vi "emballage affiche le contenu du carton_MEDIC.vi"(1 "Tableau historique":string[][](array[string])=[["MK0228606ARXA2199", "24.02.2006 11:58", "AFA", "5401/04", "1", "200"], ["MK0228606ARXA2177", "24.02.2006 12:00", "AFA", "5401/04", "1", "200"], ["MK0228606ARXA2178", "24.02.2006 12:00", "AFA", "5401/04", "1", "200"], ["MK0228606ARXA2198", "24.02.2006 12:12", "AFA", "5401/04", "1", "200"], ["MK0228606ARXA2197", "24.02.2006 12:12", "AFA", "5401/04", "1", "200"], ["MK0228606ARXA2196", "24.02.2006 12:13", "AFA", "5401/04", "1", "200"], ["MK0228606ARXA2195", "24.02.2006 12:13", "AFA", "5401/04", "1", "200"], ["MK0228606ARXA2176", "24.02.2006 12:13", "AFA", "5401/04", "1", "200"], ["MK0228606ARXA2194", "24.02.2006 12:13", "AFA", "5401/04", "1", "200"], ["MK0228606ARXA2193", "24.02.2006 12:13", "AFA", "5401/04", "1", "200"], ["MK0228606ARXA2175", "24.02.2006 12:14", "AFA", "5401/04", "1", "200"], ["MK0228606ARXA2171", "24.02.2006 12:14", "AFA", "5401/04", "1", "200"], ["MK0228606ARXA2174", "24.02.2006 12:14", "AFA", "5401/04", "1", "200"], ["MK0228606ARXA2173", "24.02.2006 12:14", "AFA", "5401/04", "1", "200"], ["MK0228606ARXA2172", "24.02.2006 12:14", "AFA", "5401/04", "1", "200"], ["MK0228606ARXA2192", "24.02.2006 12:14", "AFA", "5401/04", "1", "200"], ["MK0228606ARXA2191", "24.02.2006 12:14", "AFA", "5401/04", "1", "200"], ["MK0228606ARXA2190", "24.02.2006 12:14", "AFA", "5401/04", "1", "200"], ["MK0228606ARXA2189", "24.02.2006 12:15", "AFA", "5401/04", "1", "200"], ["MK0228606ARXA2188", "24.02.2006 12:15", "AFA", "5401/04", "1", "200"], ["MK0228606ARXB4259", "09.03.2006 17:40", "AYU", "5401/04-03.03", "5", "300"], ["MK0228606ARXB4258", "09.03.2006 17:40", "AYU", "5401/04-03.03", "5", "300"], ["MK0228606ARXB4257", "09.03.2006 17:40", "AYU", "5401/04-03.03", "5", "300"], ["MK0228606ARXB4256", "09.03.2006 17:39", "AYU", "5401/04-03.03", "5", "300"], ["MK0228606ARXB4255", "09.03.2006 17:39", "AYU", "5401/04-03.03", "5", "300"], ["MK0228606ARXB4254", "09.03.2006 17:39", "AYU", "5401/04-03.03", "5", "300"], ["MK0228606ARXB4253", "09.03.2006 17:39", "AYU", "5401/04-03.03", "5", "300"], ["MK0228606ARXB4252", "09.03.2006 17:39", "AYU", "5401/04-03.03", "5", "300"], ["MK0228606ARXB4251", "09.03.2006 17:39", "AYU", "5401/04-03.03", "5", "300"], ["MK0228606ARXB4250", "09.03.2006 17:39", "AYU", "5401/04-03.03", "5", "300"], ["MK0228606ARXB4249", "09.03.2006 17:39", "AYU", "5401/04-03.03", "5", "300"], ["MK0228606ARXB4248", "09.03.2006 17:39", "AYU", "5401/04-03.03", "5", "300"], ["MK0228606ARXB4247", "09.03.2006 17:39", "AYU", "5401/04-03.03", "5", "300"], ["MK0228606ARXB4246", "09.03.2006 17:39", "AYU", "5401/04-03.03", "5", "300"], ["MK0228606ARXB4245", "09.03.2006 17:38", "AYU", "5401/04-03.03", "5", "300"], ["MK0228606ARXB4244", "09.03.2006 17:38", "AYU", "5401/04-03.03", "5", "300"], ["MK0228606ARXB4243", "09.03.2006 17:38", "AYU", "5401/04-03.03", "5", "300"], ["MK0228606ARXB4242", "09.03.2006 17:38", "AYU", "5401/04-03.03", "5", "300"], ["MK0228606ARXB4241", "09.03.2006 17:38", "AYU", "5401/04-03.03", "5", "300"], ["MK0228606ARXB4240", "09.03.2006 17:38", "AYU", "5401/04-03.03", "5", "300"], ["MK0228606ARXB4239", "09.03.2006 17:33", "AYU", "5401/04-03.03", "4", "300"], ["MK0228606ARXB4238", "09.03.2006 17:32", "AYU", "5401/04-03.03", "4", "300"], ["MK0228606ARXB4237", "09.03.2006 17:32", "AYU", "5401/04-03.03", "4", "300"], ["MK0228606ARXB4236", "09.03.2006 17:32", "AYU", "5401/04-03.03", "4", "300"], ["MK0228606ARXB4235", "09.03.2006 17:32", "AYU", "5401/04-03.03", "4", "300"], ["MK0228606ARXB4234", "09.03.2006 17:32", "AYU", "5401/04-03.03", "4", "300"], ["MK0228606ARXB4233", "09.03.2006 17:32", "AYU", "5401/04-03.03", "4", "300"], ["MK0228606ARXB4232", "09.03.2006 17:32", "AYU", "5401/04-03.03", "4", "300"], ["MK0228606ARXB4231", "09.03.2006 17:31", "AYU", "5401/04-03.03", "4", "300"], ["MK0228606ARXB4230", "09.03.2006 17:31", "AYU", "5401/04-03.03", "4", "300"], ["MK0228606ARXB4229", "09.03.2006 17:31", "AYU", "5401/04-03.03", "4", "300"], ["MK0228606ARXB4228", "09.03.2006 17:31", "AYU", "5401/04-03.03", "4", "300"], ["MK0228606ARXB4227", "09.03.2006 17:31", "AYU", "5401/04-03.03", "4", "300"], ["MK0228606ARXB4226", "09.03.2006 17:31", "AYU", "5401/04-03.03", "4", "300"], ["MK0228606ARXB4225", "09.03.2006 17:30", "AYU", "5401/04-03.03", "4", "300"], ["MK0228606ARXB4224", "09.03.2006 17:30", "AYU", "5401/04-03.03", "4", "300"], ["MK0228606ARXB4223", "09.03.2006 17:30", "AYU", "5401/04-03.03", "4", "300"], ["MK0228606ARXB4222", "09.03.2006 17:30", "AYU", "5401/04-03.03", "4", "300"], ["MK0228606ARXB4221", "09.03.2006 17:30", "AYU", "5401/04-03.03", "4", "300"], ["MK0228606ARXB4220", "09.03.2006 17:30", "AYU", "5401/04-03.03", "4", "300"], ["MK0228606ARXB4219", "09.03.2006 17:24", "AYU", "5401/04-03.03", "3", "300"], ["MK0228606ARXB4218", "09.03.2006 17:23", "AYU", "5401/04-03.03", "3", "300"], ["MK0228606ARXB4217", "09.03.2006 17:23", "AYU", "5401/04-03.03", "3", "300"], ["MK0228606ARXB4216", "09.03.2006 17:23", "AYU", "5401/04-03.03", "3", "300"], ["MK0228606ARXB4215", "09.03.2006 17:23", "AYU", "5401/04-03.03", "3", "300"], ["MK0228606ARXB4214", "09.03.2006 17:23", "AYU", "5401/04-03.03", "3", "300"], ["MK0228606ARXB4213", "09.03.2006 17:23", "AYU", "5401/04-03.03", "3", "300"], ["MK0228606ARXB4212", "09.03.2006 17:22", "AYU", "5401/04-03.03", "3", "300"], ["MK0228606ARXB4211", "09.03.2006 17:21", "AYU", "5401/04-03.03", "3", "300"], ["MK0228606ARXB4210", "09.03.2006 17:21", "AYU", "5401/04-03.03", "3", "300"], ["MK0228606ARXB4209", "09.03.2006 17:21", "AYU", "5401/04-03.03", "3", "300"], ["MK0228606ARXB4208", "09.03.2006 17:20", "AYU", "5401/04-03.03", "3", "300"], ["MK0228606ARXB4207", "09.03.2006 17:20", "AYU", "5401/04-03.03", "3", "300"], ["MK0228606ARXB4206", "09.03.2006 17:20", "AYU", "5401/04-03.03", "3", "300"], ["MK0228606ARXB4205", "09.03.2006 17:20", "AYU", "5401/04-03.03", "3", "300"], ["MK0228606ARXB4204", "09.03.2006 17:20", "AYU", "5401/04-03.03", "3", "300"], ["MK0228606ARXB4203", "09.03.2006 17:20", "AYU", "5401/04-03.03", "3", "300"], ["MK0228606ARXB4202", "09.03.2006 17:19", "AYU", "5401/04-03.03", "3", "300"], ["MK0228606ARXB4201", "09.03.2006 17:19", "AYU", "5401/04-03.03", "3", "300"], ["MK0228606ARXB4200", "09.03.2006 17:18", "AYU", "5401/04-03.03", "3", "300"], ["MK0228606ARXB4199", "09.03.2006 17:12", "AYU", "5401/04-03.03", "2", "300"], ["MK0228606ARXB4198", "09.03.2006 17:11", "AYU", "5401/04-03.03", "2", "300"], ["MK0228606ARXB4197", "09.03.2006 17:11", "AYU", "5401/04-03.03", "2", "300"], ["MK0228606ARXB4196", "09.03.2006 17:11", "AYU", "5401/04-03.03", "2", "300"], ["MK0228606ARXB4195", "09.03.2006 17:11", "AYU", "5401/04-03.03", "2", "300"], ["MK0228606ARXB4194", "09.03.2006 17:11", "AYU", "5401/04-03.03", "2", "300"], ["MK0228606ARXB4193", "09.03.2006 17:11", "AYU", "5401/04-03.03", "2", "300"], ["MK0228606ARXB4192", "09.03.2006 17:10", "AYU", "5401/04-03.03", "2", "300"], ["MK0228606ARXB4191", "09.03.2006 17:10", "AYU", "5401/04-03.03", "2", "300"], ["MK0228606ARXB4190", "09.03.2006 17:10", "AYU", "5401/04-03.03", "2", "300"], ["MK0228606ARXB4189", "09.03.2006 17:10", "AYU", "5401/04-03.03", "2", "300"], ["MK0228606ARXB4188", "09.03.2006 17:10", "AYU", "5401/04-03.03", "2", "300"], ["MK0228606ARXB4187", "09.03.2006 17:10", "AYU", "5401/04-03.03", "2", "300"], ["MK0228606ARXB4186", "09.03.2006 17:10", "AYU", "5401/04-03.03", "2", "300"], ["MK0228606ARXB4185", "09.03.2006 17:10", "AYU", "5401/04-03.03", "2", "300"], ["MK0228606ARXB4184", "09.03.2006 17:09", "AYU", "5401/04-03.03", "2", "300"], ["MK0228606ARXB4183", "09.03.2006 17:09", "AYU", "5401/04-03.03", "2", "300"], ["MK0228606ARXB4182", "09.03.2006 17:09", "AYU", "5401/04-03.03", "2", "300"], ["MK0228606ARXB4181", "09.03.2006 17:08", "AYU", "5401/04-03.03", "2", "300"], ["MK0228606ARXB4180", "09.03.2006 17:08", "AYU", "5401/04-03.03", "2", "300"], ["MK0228606ARXB4179", "09.03.2006 17:01", "AYU", "5401/04-03.03", "1", "300"], ["MK0228606ARXB4178", "09.03.2006 17:01", "AYU", "5401/04-03.03", "1", "300"], ["MK0228606ARXB4177", "09.03.2006 17:01", "AYU", "5401/04-03.03", "1", "300"], ["MK0228606ARXB4176", "09.03.2006 17:01", "AYU", "5401/04-03.03", "1", "300"], ["MK0228606ARXB4175", "09.03.2006 17:00", "AYU", "5401/04-03.03", "1", "300"], ["MK0228606ARXB4174", "09.03.2006 17:00", "AYU", "5401/04-03.03", "1", "300"], ["MK0228606ARXB4173", "09.03.2006 17:00", "AYU", "5401/04-03.03", "1", "300"], ["MK0228606ARXB4172", "09.03.2006 17:00", "AYU", "5401/04-03.03", "1", "300"], ["MK0228606ARXB4171", "09.03.2006 17:00", "AYU", "5401/04-03.03", "1", "300"], ["MK0228606ARXB4170", "09.03.2006 16:57", "AYU", "5401/04-03.03", "1", "300"], ["MK0228606ARXB4169", "09.03.2006 16:57", "AYU", "5401/04-03.03", "1", "300"], ["MK0228606ARXB4168", "09.03.2006 16:56", "AYU", "5401/04-03.03", "1", "300"], ["MK0228606ARXB4167", "09.03.2006 16:56", "AYU", "5401/04-03.03", "1", "300"], ["MK0228606ARXB4166", "09.03.2006 16:56", "AYU", "5401/04-03.03", "1", "300"], ["MK0228606ARXB4165", "09.03.2006 16:55", "AYU", "5401/04-03.03", "1", "300"], ["MK0228606ARXB4164", "09.03.2006 16:55", "AYU", "5401/04-03.03", "1", "300"], ["MK0228606ARXB4163", "09.03.2006 16:55", "AYU", "5401/04-03.03", "1", "300"], ["MK0228606ARXB4162", "09.03.2006 16:54", "AYU", "5401/04-03.03", "1", "300"], ["MK0228606ARXB4161", "09.03.2006 16:54", "AYU", "5401/04-03.03", "1", "300"], ["MK0228606ARXB4160", "09.03.2006 16:52", "AYU", "5401/04-03.03", "1", "300"], ["MK0228606ARXB4158", "10.03.2006 08:35", "AYU", "5401/04-03.03", "1", "300"], ["MK0228606ARXB4159", "10.03.2006 08:34", "AYU", "5401/04-03.03", "1", "300"]], 2 "chaîne 2D emballage en cours":string) -> ()   [LabVIEW 2020]
panel:
  in  "Tableau":string[](array[string])
  in  "quitter":bool
  out "Piéces dans le carton":i32(listbox)
  out "Numéro de la commande :":string
  in  "numéro du carton :":i16
  # "(si rien : prend la liste en cours d'emballage)"
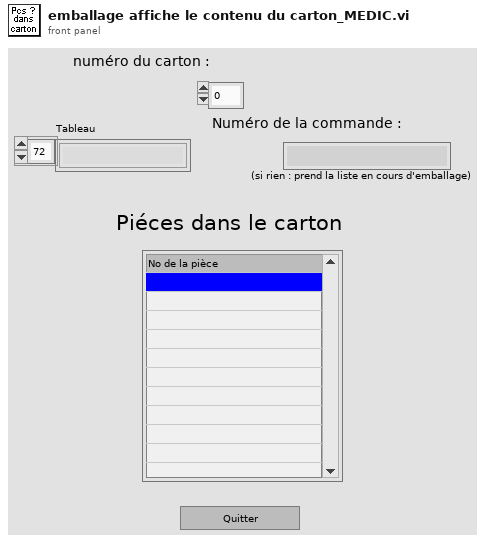
[diagram p1: front panel]
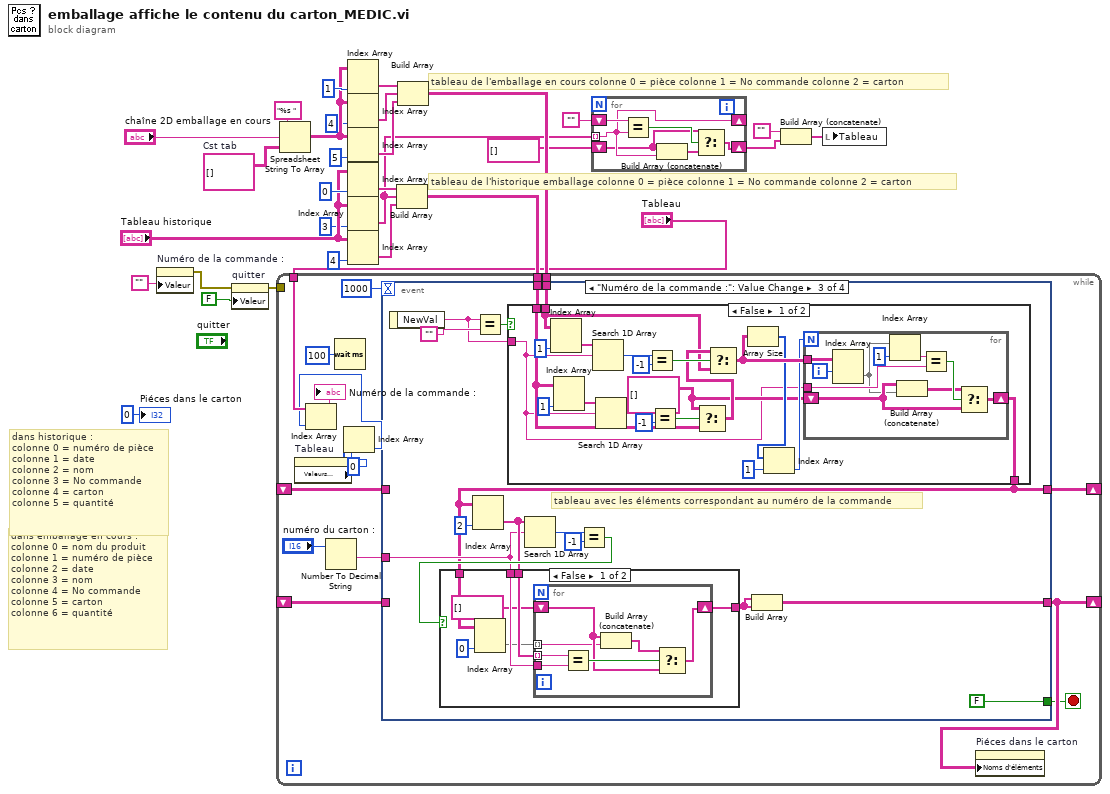
[diagram p0: block diagram]
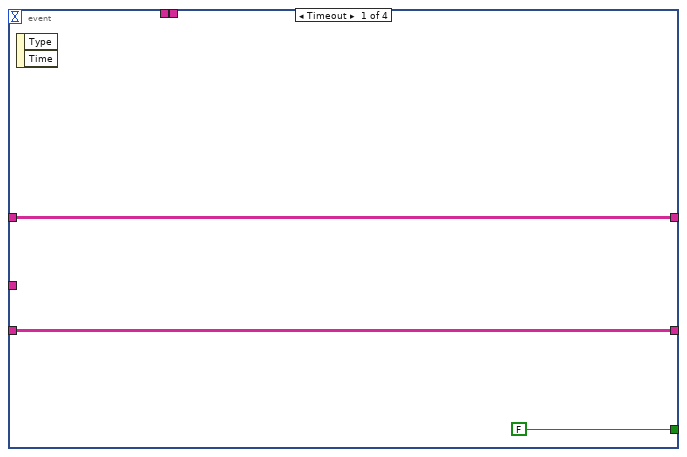
[diagram p2: hidden frame]
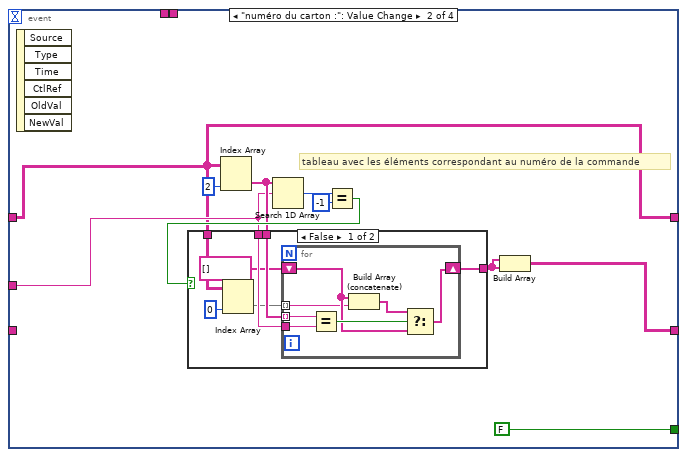
[diagram p3: hidden frame]
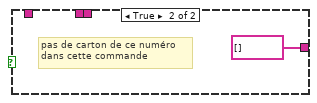
[diagram p4: hidden frame]
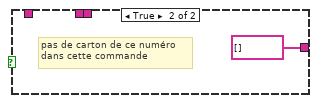
[diagram p5: hidden frame]
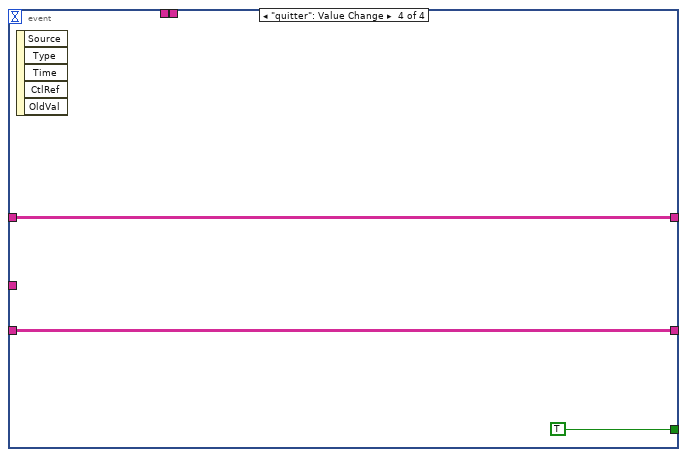
[diagram p7: hidden frame]
diagram:
  w25 = string[][] []  # Cst tab
  # "tableau de l'historique emballage colonne 0 = pièce colonne 1 = No commande colonne 2 = carton"
  # "tableau de l'emballage en cours colonne 0 = pièce colonne 1 = No commande colonne 2 = carton"
  # "dans emballage en cours :\ncolonne 0 = nom du produit\ncolonne 1 = numéro de pièce\ncolonne 2 = date\ncolonne 3 = nom\ncolonne 4 = No commande\ncolonne 5 = carton\ncolonne 6 = quantité"
  # "dans historique :\ncolonne 0 = numéro de pièce\ncolonne 1 = date\ncolonne 2 = nom\ncolonne 3 = No commande\ncolonne 4 = carton\ncolonne 5 = quantité"
  n1 = property on="Numéro de la commande :" class="Str"("Valeur"="") -> (error out=w21:errorcluster)  [unwired: 2 in, 1 out]
  n2 = property on="quitter" class="Bool (strict)"(error in=w21, "Valeur"=FALSE) -> (error out=w29:errorcluster)  [unwired: 1 in, 1 out]
  n3 = Spreadsheet String To Array(format string="%s ", spreadsheet string="chaîne 2D emballage en cours", array type (2D Dbl)=w25) -> (array=w16:string[][])  [unwired: 1 in]
  n4 = Index Array(array=w16, index (col)=1) -> (element=w22:string[])  [unwired: 1 in]
  n5 = Index Array(array=w16, index (col)=4) -> (element=w8:string[])  [unwired: 1 in]
  n6 = Index Array(array=w16, index (col)=5) -> (element=w12:string[])  [unwired: 1 in]
  n7 = Index Array(array="Tableau historique", index (col)=0) -> (element=w17:string[])  [unwired: 1 in]
  n8 = Index Array(array="Tableau historique", index (col)=3) -> (element=w5:string[])  [unwired: 1 in]
  n9 = Index Array(array="Tableau historique", index (col)=4) -> (element=w11:string[])  [unwired: 1 in]
  n10 = Build Array(w17, w5, w11) -> (w10:string[][])
  n11 = Build Array(w22, w8, w12) -> (w9:string[][])
  n12 = while {
    tunnel: w29 -> [_]
    tunnel: w10 -> [w39]
    tunnel: w9 -> [w40]
    shift-right: [w42] -> _
    shift-left: _ -> [w43]
    shift-right: [w37] -> _
    shift-left: _ -> [w36]
    tunnel: "Tableau" -> [w35]
    stop <- w41 stop-if-true
    n13 = property on="Tableau" class="Arr (strict)"() -> ("Valeurs d'indice"=w33:u32[])  [unwired: 2 in, 2 out]
    n14 = Number To Decimal String(number="numéro du carton :") -> (decimal integer string=w46:string)  [unwired: 1 in]
    n15 = Wait (ms)(milliseconds to wait=100) -> ()  [unwired: 1 out]
    n16 = Index Array(array=w33, index=0) -> (element=w32:u32)
    n17 = Index Array(array=w35, index=w32) -> (element=→"Numéro de la commande :":string)
    n18 = event shown="[2] \"Numéro de la commande :\": Value Change" {
      selector: _ -> [_ _ _ _]
      dyn-events: _ -> [_ _ _ _]
      timeout: 1000 -> [_ _ _ _]
      tunnel: w46 -> [_ w53 w81 _]
      tunnel: [w47 w51 w80 w136] -> w37
      tunnel: [FALSE FALSE FALSE TRUE] -> w41
      tunnel: [w48 w50 w77 w137] -> w42
      tunnel: w43 -> [w48 _ _ w137]
      tunnel: w40 -> [_ _ w76 _]
      tunnel: w39 -> [_ _ w75 _]
      tunnel: w36 -> [w47 w51 _ w136]
      event Timeout {
        n19 = event-data() -> ()  [unwired: 1 in, 2 out]
      }
      event "numéro du carton :": Value Change {
        # "tableau avec les éléments correspondant au numéro de la commande"
        n20 = event-data() -> ()  [unwired: 1 in, 6 out]
        n21 = Index Array(array=w51, index (col)=2) -> (element=w57:string[])  [unwired: 1 in]
        n22 = Search 1D Array(1D array=w57, element=w53) -> (index of element=w55:i32)  [unwired: 1 in]
        n23 = Equal?(x=w55, y=-1) -> (x = y?=w59:bool)
        n24 = case shown="False" w59 {
          tunnel: w57 -> [w66 _]
          tunnel: w53 -> [w65 _]
          tunnel: [w63 string[] []] -> w58
          tunnel: w51 -> [w61 _]
          frame False {
            n25 = Index Array(array=w61, index (col)=0) -> (element=w60:string[])  [unwired: 1 in]
            n26 = for {
              tunnel: w66 -> [w69] mode=indexing
              tunnel: w65 -> [w73]
              shift-right: [w71] -> w63
              shift-left: string[] [] -> [w70]
              tunnel: w60 -> [w67] mode=indexing
              n27 = Equal?(x=w69, y=w73) -> (x = y?=w72:bool)
              n28 = Build Array (concatenate)(w70, w67) -> (w68:string[])
              n29 = Select(t=w68, s=w72, f=w70) -> (s? t:f=w71:string[])
            }
          }
          frame True {
            # "pas de carton de ce numéro \ndans cette commande"
          }
        }
        n30 = Build Array(w58, w58) -> (w50:string[][])
      }
      event "Numéro de la commande :": Value Change {
        # "tableau avec les éléments correspondant au numéro de la commande"
        n31 = event-data() -> ("NewVal"=w79:string)  [unwired: 1 in]
        n32 = Equal?(x=w79, y="") -> (x = y?=w88:bool)
        n33 = case shown="False" w88 {
          tunnel: w76 -> [w105 w135]
          tunnel: w79 -> [w107 _]
          tunnel: w75 -> [w113 _]
          tunnel: [w106 w135] -> w80
          frame False {
            w108 = string[][] []
            n34 = Index Array(array=w105, index (col)=1) -> (element=w121:string[])  [unwired: 1 in]
            n35 = Index Array(array=w113, index (col)=1) -> (element=w120:string[])  [unwired: 1 in]
            n36 = Search 1D Array(1D array=w121, element=w107) -> (index of element=w123:i32)  [unwired: 1 in]
            n37 = Search 1D Array(1D array=w120, element=w107) -> (index of element=w118:i32)  [unwired: 1 in]
            n38 = Equal?(x=w123, y=-1) -> (x = y?=w116:bool)
            n39 = Equal?(x=w118, y=-1) -> (x = y?=w114:bool)
            n40 = Select(t=w108, s=w114, f=w113) -> (s? t:f=w115:string[][])
            n41 = Select(t=w115, s=w116, f=w105) -> (s? t:f=w112:string[][])
            n42 = Array Size(array=w112) -> (size(s)=w111:i32[])
            n43 = Index Array(array=w111, index=1) -> (element=w109:i32)
            n44 = for {
              N: w109 -> [_]
              tunnel: w112 -> [w133]
              shift-right: [w134] -> w106
              shift-left: w108 -> [w127]
              tunnel: w107 -> [w130]
              i -> [w132]
              n45 = Index Array(array=w133, index (row)=w132) -> (element=w126:string[])  [unwired: 1 in]
              n46 = Index Array(array=w126, index=1) -> (element=w131:string)
              n47 = Build Array (concatenate)(w127, w126) -> (w125:string[][])
              n48 = Equal?(x=w131, y=w130) -> (x = y?=w129:bool)
              n49 = Select(t=w125, s=w129, f=w127) -> (s? t:f=w134:string[][])
            }
          }
          frame True {
            # "No commande =\"\" => commande en cours"
          }
        }
        n50 = Index Array(array=w80, index (col)=2) -> (element=w85:string[])  [unwired: 1 in]
        n51 = Search 1D Array(1D array=w85, element=w81) -> (index of element=w83:i32)  [unwired: 1 in]
        n52 = Equal?(x=w83, y=-1) -> (x = y?=w87:bool)
        n53 = case shown="False" w87 {
          tunnel: w85 -> [w96 _]
          tunnel: w81 -> [w95 _]
          tunnel: [w93 string[] []] -> w86
          tunnel: w80 -> [w91 _]
          frame False {
            n54 = Index Array(array=w91, index (col)=0) -> (element=w90:string[])  [unwired: 1 in]
            n55 = for {
              tunnel: w96 -> [w99] mode=indexing
              tunnel: w95 -> [w103]
              shift-right: [w101] -> w93
              shift-left: string[] [] -> [w100]
              tunnel: w90 -> [w97] mode=indexing
              n56 = Equal?(x=w99, y=w103) -> (x = y?=w102:bool)
              n57 = Build Array (concatenate)(w100, w97) -> (w98:string[])
              n58 = Select(t=w98, s=w102, f=w100) -> (s? t:f=w101:string[])
            }
          }
          frame True {
            # "pas de carton de ce numéro \ndans cette commande"
          }
        }
        n59 = Build Array(w86, w86) -> (w77:string[][])
      }
      event "quitter": Value Change {
        n60 = event-data() -> ()  [unwired: 1 in, 5 out]
      }
    }
    n61 = property on="Piéces dans le carton" class="MCListbox (strict)"("Noms d'éléments"=w42) -> ()  [unwired: 2 in, 2 out]
  }
  n62 = for {
    tunnel: w5 -> [w143] mode=indexing
    shift-right: [w143] -> _
    shift-left: "" -> [w144]
    shift-right: [w139] -> w2
    shift-left: string[] [] -> [w141]
    n63 = Equal?(x=w144, y=w143) -> (x = y?=w142:bool)
    n64 = Build Array (concatenate)(w141, w143) -> (w140:string[])
    n65 = Select(t=w141, s=w142, f=w140) -> (s? t:f=w139:string[])
  }
  n66 = Build Array (concatenate)("", w2) -> (w1:string[])
  n67 = local write "Tableau"(w1) -> ()
  "Piéces dans le carton" <- 0
